vi "Draw Wheel Outline.vi"(4 "angle (rad)":dbl, 6 "color (black)":u32(colorbox), 7 "picture info":T1={"picture size"={"Width"=500, "Height"=500}, "pixels per unit"=10.0}, 8 "size":cluster{"radius":dbl, "width":dbl}, 9 "offset from center":cluster{"x":dbl, "y":dbl}, 10 "global wheel position":cluster{"x":dbl, "y":dbl}, 11 "picture in":picture) -> (3 "picture out":picture)   [LabVIEW 2017, in "NI_Robotics_Steering Picture.lvlib"]
uses:
  <vilib>/robotics/Utilities/Visualization/Steering Visualization/Steering Picture/NI_Robotics_Steering Picture.lvlib
  <vilib>/robotics/Utilities/Visualization/Steering Visualization/Steering Picture/Picture Info.ctl
  <vilib>/Utility/miscctls.llb/LVBoundsTypeDef.ctl
  <vilib>/Analysis/coordinate.llb/2D Cartesian Coordinate Rotation (Array).vi
  <vilib>/Analysis/NI_AALPro.lvlib
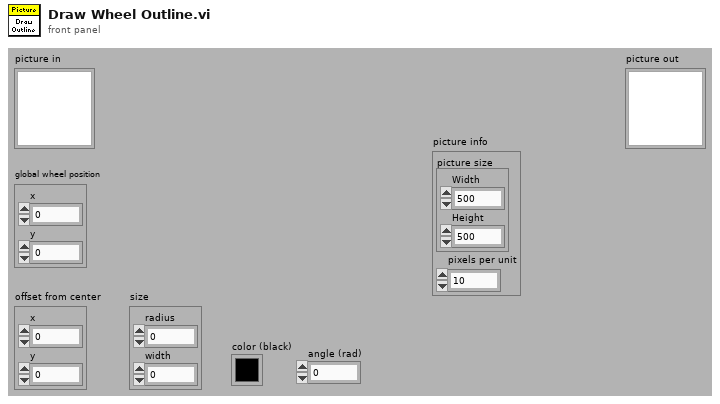
[diagram p1: front panel]
types:
  T1 = typedef "NI_Robotics_Steering Picture.lvlib/Picture Info.ctl" = cluster{"picture size":T2, "pixels per unit":dbl}
  T2 = typedef "LVBoundsTypeDef.ctl" = cluster{"Width":u32, "Height":u32}
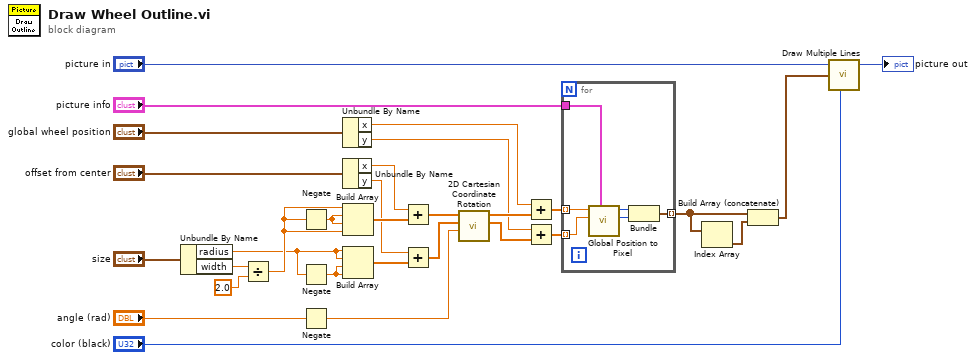
[diagram p0: block diagram]
diagram:
  n1 = Unbundle By Name("size") -> ("radius"=w25:dbl, "width"=w29:dbl)
  n2 = Divide(x=w29, y=2.0) -> (x/y=w27:dbl)
  n3 = Negate(x=w27) -> (-x=w26:dbl)
  n4 = Negate(x=w25) -> (-x=w24:dbl)
  n5 = Negate(x="angle (rad)") -> (-x=w15:dbl)
  n6 = Unbundle By Name("global wheel position") -> ("x"=w12:dbl, "y"=w10:dbl)
  n7 = Unbundle By Name("offset from center") -> ("x"=w21:dbl, "y"=w19:dbl)
  n8 = Build Array(w27, w26, w26, w27) -> (w22:dbl[])
  n9 = Build Array(w25, w25, w24, w24) -> (w20:dbl[])
  n10 = Add(x=w21, y=w22) -> (x+y=w18:dbl[])
  n11 = Add(x=w19, y=w20) -> (x+y=w17:dbl[])
  n12 = call-poly <vilib>:"2D Cartesian Coordinate Rotation.vi"("theta"=w15, "Y"=w17, "X"=w18) -> ("Y Out"=w11:dbl[], "X Out"=w14:dbl[])  [unwired: 6 in, 1 out]
  n13 = Add(x=w12, y=w14) -> (x+y=w9:dbl[])
  n14 = Add(x=w10, y=w11) -> (x+y=w8:dbl[])
  n15 = for {
    tunnel: w9 -> [w36] mode=indexing
    tunnel: w8 -> [w35] mode=indexing
    tunnel: "picture info" -> [w34]
    tunnel: [w31] -> w7 mode=indexing
    n16 = call <vilib>:"Global Position to Pixel.vi"("picture info"=w34, "global y"=w35, "global x"=w36) -> ("pixel y"=w32:i16, "pixel x"=w33:i16)  [unwired: 7 in]
    n17 = Bundle("pixel x"=w33, "pixel y"=w32) -> (w31:cluster{"pixel x":i16, "pixel y":i16})  [unwired: 1 in]
  }
  n18 = Index Array(array=w7) -> (element=w6:cluster{"pixel x":i16, "pixel y":i16})  [unwired: 1 in]
  n19 = Build Array (concatenate)(w7, w6) -> (w4:cluster{"pixel x":i16, "pixel y":i16}[])
  n20 = call <vilib>:"Draw Multiple Lines.vi"("picture"="picture in", "line endpoints"=w4, "color(black)"="color (black)") -> ("new picture"=→"picture out":picture)  [unwired: 6 in]
